vi "Error handler.vi"(8 "error in (no error)":errorcluster, 11 "Queue in":refnum<queue>) -> (0 "error out":errorcluster)   [LabVIEW 2018]
uses:
  Message Queue/Message Cluster.ctl
  Message Queue/Message Queue.lvlib
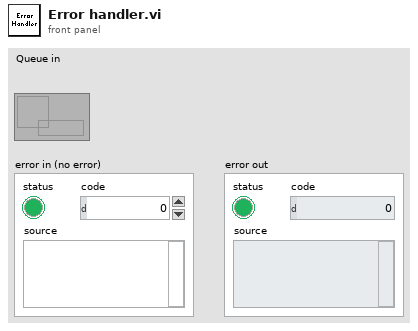
[diagram p1: front panel]
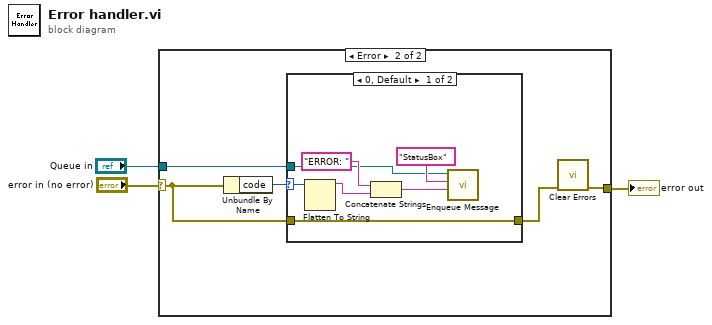
[diagram p0: block diagram]
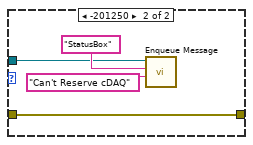
[diagram p3: hidden frame]
diagram:
  n1 = case shown="Error" "error in (no error)" {
    selector: "error in (no error)" -> [w4 w7]
    tunnel: [w4 w6] -> w3
    tunnel: "Queue in" -> [_ w8]
    frame No Error {
    }
    frame Error {
      n2 = Unbundle By Name(w7) -> ("code"=w9:i32)
      n3 = case shown="0, Default" w9 {
        selector: w9 -> [w15 _]
        tunnel: w8 -> [w11 w18]
        tunnel: w7 -> [w10 w17]
        tunnel: [w10 w17] -> w5
        frame 0, Default {
          n4 = Flatten To String(anything=w15) -> (data string=w13:string)  [unwired: 3 in, 2 out]
          n5 = Concatenate Strings("ERROR: " ("Ready..."), w13) -> (w12:string)
          n6 = call "Enqueue Message.vi"("Message Data"=w12, "Message"="StatusBox", "Message Queue"=w11) -> ()  [unwired: 7 in, 2 out]
        }
        frame -201250 {
          n7 = call "Enqueue Message.vi"("Message Data"="Can't Reserve cDAQ" ("Ready..."), "Message"="StatusBox", "Message Queue"=w18) -> ()  [unwired: 7 in, 2 out]
        }
      }
      n8 = call <vilib>:"Clear Errors.vi"("error in (no error)"=w5) -> ("error out"=w6:errorcluster)  [unwired: 5 in, 1 out]
    }
  }
  "error out" <- w3
